vi "3pt Mov Avg.vi"(10 "Value in":dbl) -> (2 "Value out":dbl)   [LabVIEW 2014]
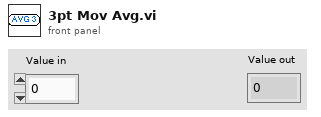
[diagram p1: front panel]
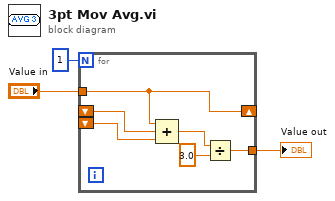
[diagram p0: block diagram]
diagram:
  n1 = for {
    N: 1 -> [_]
    tunnel: "Value in" -> [w9]
    shift-right: [w9] -> _
    shift-left: _ -> [w8]
    shift-left: _ -> [w7]
    tunnel: [w4] -> w1
    n2 = Compound Arithmetic op=ADD(w9, w8, w7) -> (w6:dbl)
    n3 = Divide(x=w6, y=3.0) -> (x/y=w4:dbl)
  }
  "Value out" <- w1
